vi "Get UDL File Path.vi"() -> (0 "connection information":string)   [LabVIEW 2015]
doc: "This VI is used as a subVI in all the Database Tools example VIs. This VI looks for a file in the Examples/database directory called LabVIEW.udl and returns the path. \n\nA UDL (Universal Data Link) file specifies the connection to an OLE DB provider and a data source. The LabVIEW.udl supplied with the Database Tools examples specifies the Microsoft Jet 4.0 OLE DB Provider connected to the database file named LabVIEW.mdb."
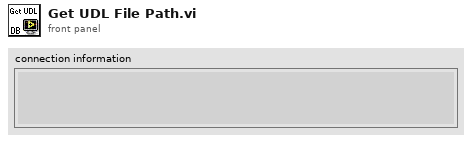
[diagram p1: front panel]
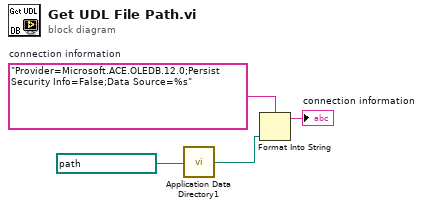
[diagram p0: block diagram]
diagram:
  w4 = "Provider=Microsoft.ACE.OLEDB.12.0;Persist Security Info=False;Data Source=%s"  # connection information
  n1 = call "Application Data Directory1.vi"("Relative path (.)"=path "热敏电阻.accdb") -> ("Application Directory (+ Relative)"=w1:path)
  n2 = Format Into String(format string=w4, w1) -> (resulting string=→"connection information":string)  [unwired: 2 in, 1 out]
